vi "Close.vi"(8 "error in":errorcluster, 11 "Thermometer DAQmx RTD Cont CFG in":refnum<class "Thermometer DAQmx RTD Cont CFG.lvclass">) -> (0 "error out":errorcluster, 3 "Thermometer DAQmx RTD Cont CFG out":refnum<class "Thermometer DAQmx RTD Cont CFG.lvclass">)   [LabVIEW 2024, in "Thermometer DAQmx RTD Cont CFG.lvclass"]
uses:
  Thermometer DAQmx RTD Cont CFG.lvclass
  Thermometer DAQmx RTD Cont CFG.lvclass/Thermometer DAQmx RTD Cont CFG.ctl
  DAQmx Base CFG/DAQmx Base CFG.lvclass
  Buffers/BufferLossless/BufferLossless.lvclass
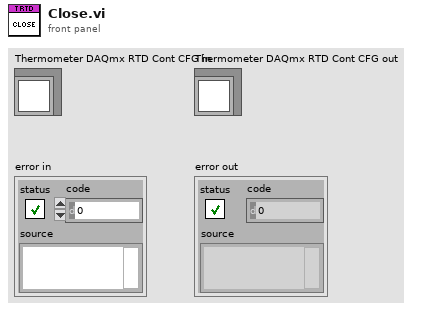
[diagram p1: front panel]
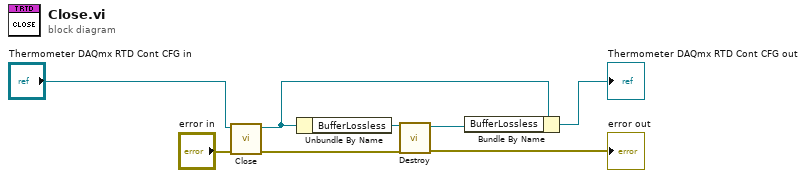
[diagram p0: block diagram]
diagram:
  n1 = call-parent "Close.vi"("error in"="error in", "DAQmx Base CFG in"="Thermometer DAQmx RTD Cont CFG in") -> ("error out"=w5:errorcluster, "DAQmx Base CFG out"=w2:refnum<class "Thermometer DAQmx RTD Cont CFG.lvclass">)  [unwired: 8 in]
  n2 = Unbundle By Name(w2) -> ("BufferLossless"=w6:refnum<class "BufferLossless.lvclass">)
  n3 = call "Destroy.vi"("error in"=w5, "BufferLossless in"=w6) -> ("error out"=→"error out":errorcluster, "BufferLossless out"=w3:refnum<class "BufferLossless.lvclass">)  [unwired: 8 in]
  n4 = Bundle By Name(cluster=w2, "BufferLossless"=w3) -> (→"Thermometer DAQmx RTD Cont CFG out":refnum<class "Thermometer DAQmx RTD Cont CFG.lvclass">)
